vi "Configure Measurement.vi"(5 "Trigger Offset Points (0)":i32, 6 "Sample Interval (20.48e-6)":dbl=2.048e-05 format="%^.3e", 7 "Points (1024)":i32=1024, 8 "error in (no error)":errorcluster {"code" format="%.0x"}, 9 "Measurement Type (1: Voltage)":i32(ring)=1 items=["Voltage"=1, "Current"=0], 10 "Channel Name (1)":string="1", 11 "VISA resource name":refnum<visa-resource-name>) -> (0 "error out":errorcluster {"code" format="%.0x"}, 3 "VISA resource name out":refnum<visa-resource-name>)   [LabVIEW 2018, in "Agilent N6700 Series.lvlib"]
doc: "Sets the trigger offset points, the sweep points, the sample interval, and the measurement functions. \n\n<b>Note:</b>\nMeasurement Type is ignored when programming Models N6761A and N6762A. This is because these models measure both voltage and current simultaneously."
uses:
  Agilent N6700 Series.lvlib
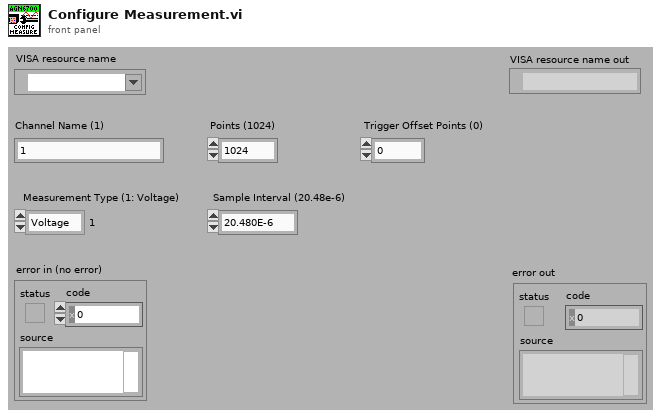
[diagram p1: front panel]
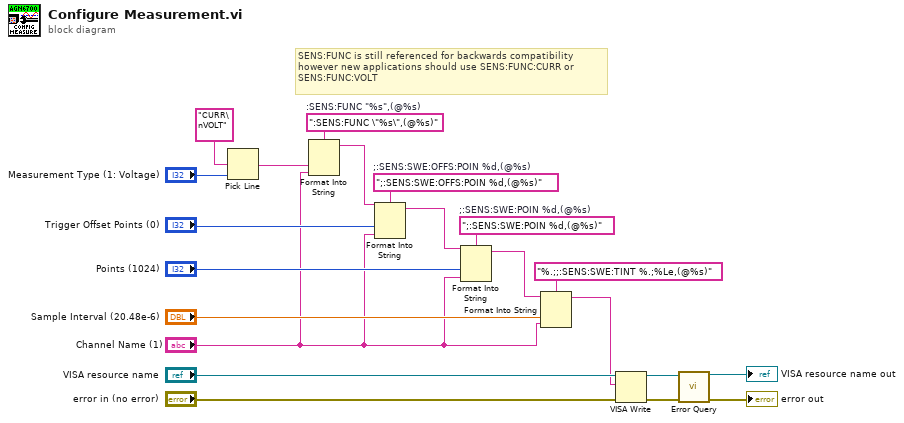
[diagram p0: block diagram]
diagram:
  w14 = ";:SENS:SWE:OFFS:POIN %d,(@%s)"  # ;:SENS:SWE:OFFS:POIN %d,(@%s)
  w16 = ":SENS:FUNC \"%s\",(@%s)"  # :SENS:FUNC "%s",(@%s)
  w21 = ";:SENS:SWE:POIN %d,(@%s)"  # ;:SENS:SWE:POIN %d,(@%s)
  # "SENS:FUNC is still referenced for backwards compatibility\nhowever new applications should use SENS:FUNC:CURR or\nSENS:FUNC:VOLT"
  n1 = Pick Line(multi-line string="CURR\nVOLT", line index="Measurement Type (1: Voltage)") -> (output string=w15:string)  [unwired: 1 in]
  n2 = Format Into String(format string=w16, w15, "Channel Name (1)") -> (resulting string=w6:string)  [unwired: 2 in, 1 out]
  n3 = Format Into String(format string=w14, initial string=w6, "Trigger Offset Points (0)", "Channel Name (1)") -> (resulting string=w7:string)  [unwired: 1 in, 1 out]
  n4 = Format Into String(format string=w21, initial string=w7, "Points (1024)", "Channel Name (1)") -> (resulting string=w8:string)  [unwired: 1 in, 1 out]
  n5 = Format Into String(format string="%.;;:SENS:SWE:TINT %.;%Le,(@%s)", initial string=w8, "Sample Interval (20.48e-6)", "Channel Name (1)") -> (resulting string=w9:string)  [unwired: 1 in, 1 out]
  n6 = VISA Write(VISA resource name="VISA resource name", write buffer=w9, error in (no error)="error in (no error)") -> (VISA resource name out=w2:refnum<visa-resource-name>, error out=w1:errorcluster)  [unwired: 1 out]
  n7 = call "Error Query.vi"("VISA resource name"=w2, "error in (no error)"=w1) -> ("VISA resource name out"=→"VISA resource name out":refnum<visa-resource-name>, "error out"=→"error out":errorcluster)  [unwired: 10 in, 2 out]
